vi "WSVCAP SHL Host TL I2C Write.vi"(0 "C1 Data Out":u8[][](array[numeric]) format="%.0x", 5 "C2 Data Out":u8[][](array[numeric]) format="%.0x", 7 "C3 Data Out":u8[][](array[numeric]) format="%.0x", 9 "Socket Mask [U64]":u64=1 format="%012x", 11 "error in":errorcluster, 12 "Sub Address":u8=20, 13 "Log (T)":bool=TRUE) -> (15 "error out":errorcluster)   [LabVIEW 2012]
uses:
  Type Defs/WSVCAP SHL Function Enum.ctl
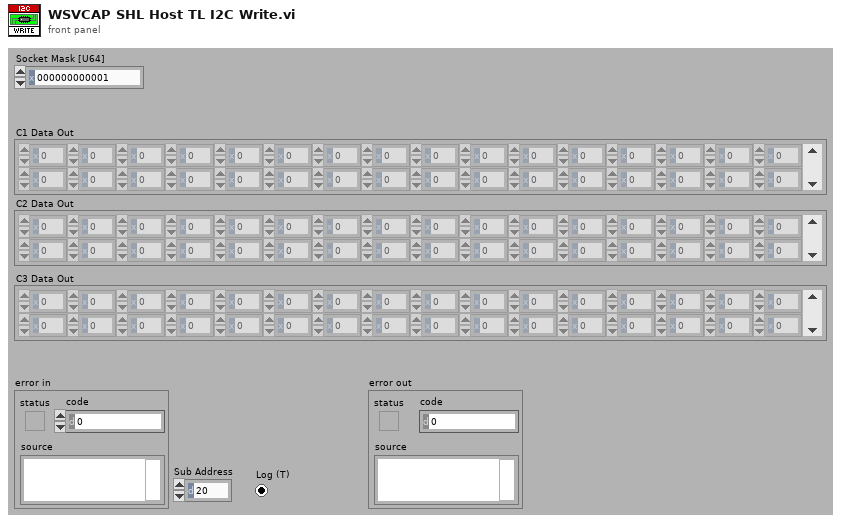
[diagram p1: front panel]
types:
  T1 = typedef "WSVCAP SHL Function Enum.ctl" = enum16{"Initialize", "Configure I2C", "Configure SPI", "Configure RFFE", "Write I2C", "Read I2C", "Write/Read SPI", "Start SPI Cycle", "Stop SPI Cycle", "Write RFFE", "Read RFFE", "Start RFFE Cycle", "Stop RFFE Cycle", "Get Status", "Close"}
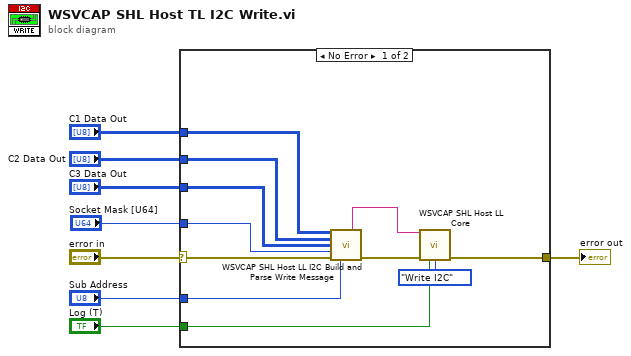
[diagram p0: block diagram]
diagram:
  n1 = case shown="No Error" "error in" {
    selector: "error in" -> [w17 w20]
    tunnel: [w18 w20] -> w8
    tunnel: "C1 Data Out" -> [w12 _]
    tunnel: "C2 Data Out" -> [w11 _]
    tunnel: "Sub Address" -> [w10 _]
    tunnel: "Socket Mask [U64]" -> [w14 _]
    tunnel: "Log (T)" -> [w13 _]
    tunnel: "C3 Data Out" -> [w9 _]
    frame No Error {
      n2 = call "WSVCAP SHL Host LL I2C Build and Parse Write Message.vi"("C1 Write Data In [DUT Ordered]"=w12, "C2 Write Data [DUT Ordered]"=w11, "C3Write Data [DUT Ordered]"=w9, "Socket Mask [U64] In"=w14, "error in"=w17, "Sub Address In"=w10) -> ("Message Out"=w15:string, "error out"=w16:errorcluster)  [unwired: 3 in, 5 out]
      n3 = call "WSVCAP SHL Host LL Core.vi"("Message In"=w15, "error in"=w16, "Log (T)"=w13, "Function"=WSVCAP_SHL_Function_Enum."Write I2C") -> ("error out"=w18:errorcluster)  [unwired: 9 in, 2 out]
    }
    frame Error {
    }
  }
  "error out" <- w8
